vi "LoopselFF.VI"() -> ()   [LabVIEW 2015]
panel:
  in  "alloc mem":bool
  out "FREE \nRAM MB":u64=14006
  out "BUILT-IN\nRAM MB":u64=16662
  out "SEC":dbl=0.06
  out "MB RAM":u64=6
  in  "pos slope":u8=1
  in  "both slopes":u8
  in  "DAT in 10ns":u32
  out "FIFO overflow":bool
  in  "extTrig 0/1":u8
  in  "stop all":bool
  in  "start new block":bool
  in  "Slide":u32(slide)=27666 scale=1.0..3000.0
  in  "frequency[Hz]":u32
  in  "no.of samples (nos)":u32=3000
  in  "exposuretime[ms]":dbl=0.02 format="%.3f"
  out "Signalverlaufgraph":u16[](graph)
  # "Start with run"
  # "Abort with ESC"
  # "1x"
  # "repeat"
  # "exit here"
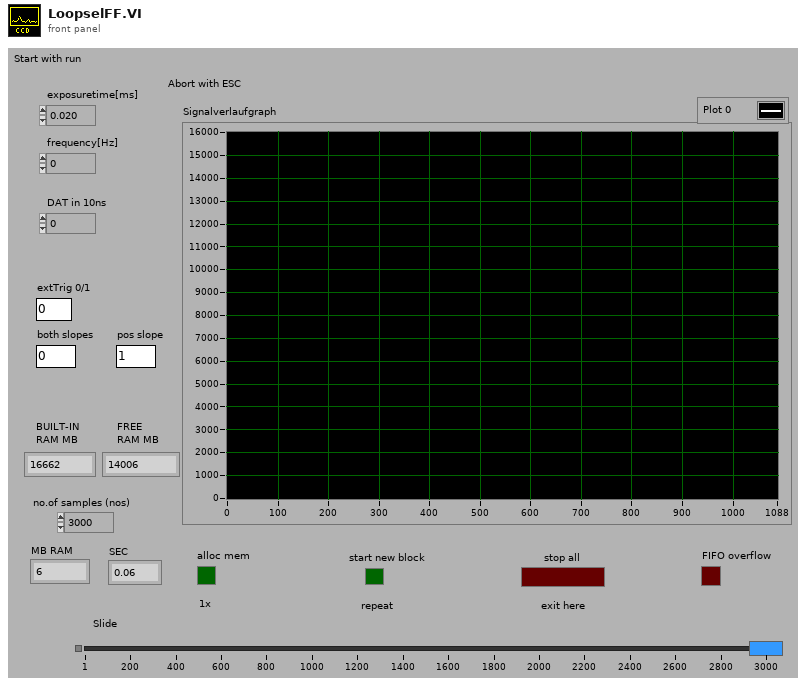
[diagram p1: front panel]
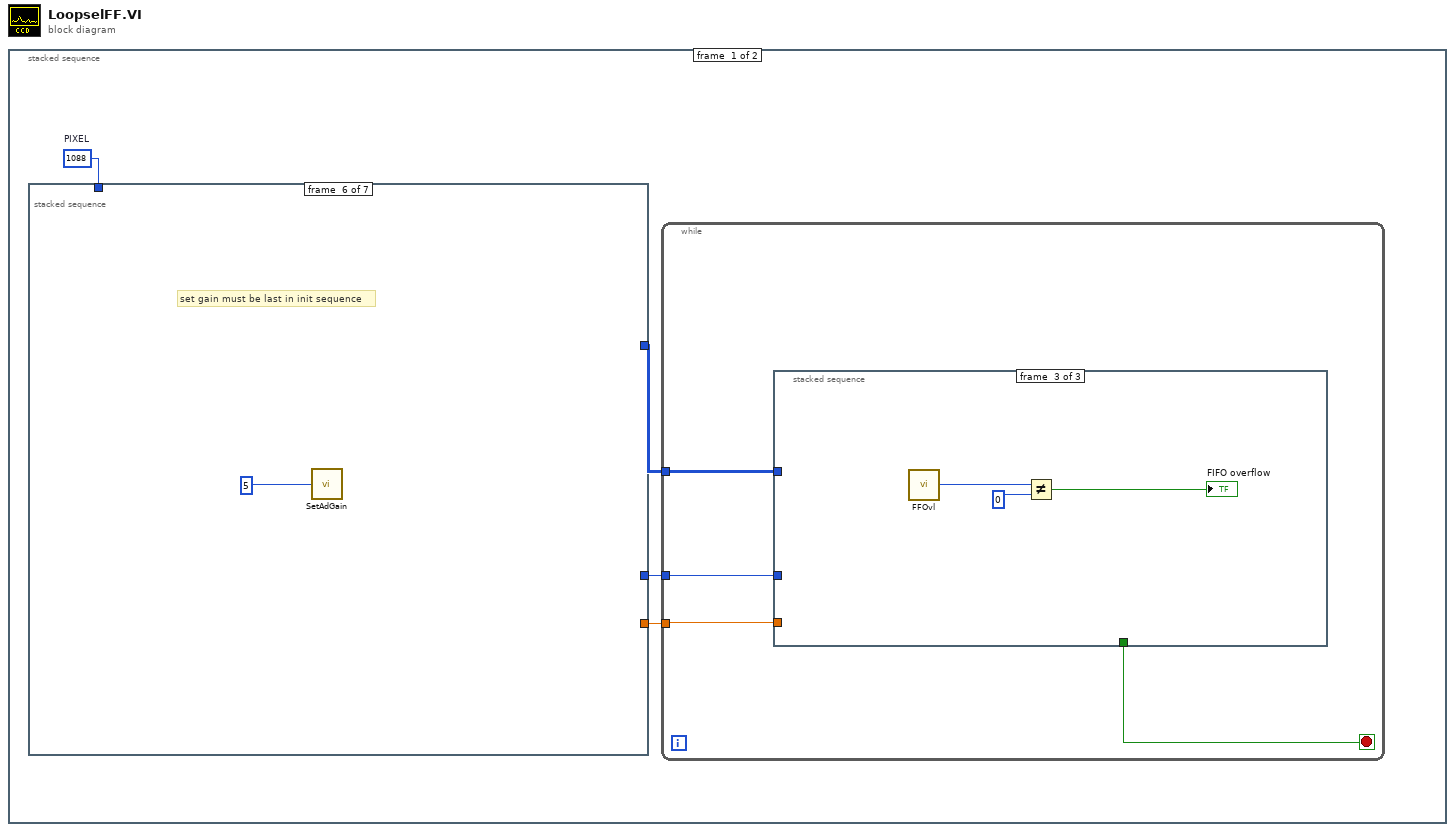
[diagram p0: block diagram]
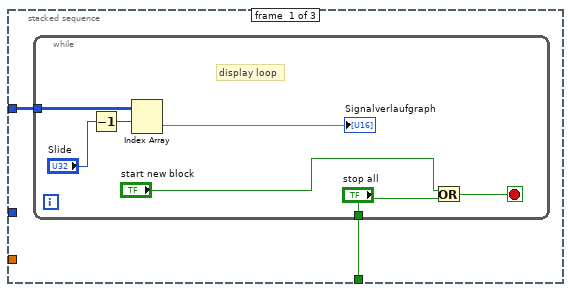
[diagram p2: hidden frame]
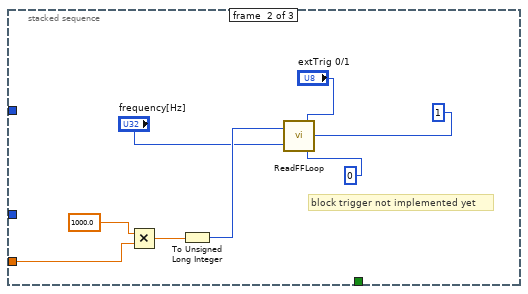
[diagram p3: hidden frame]
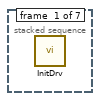
[diagram p4: hidden frame]
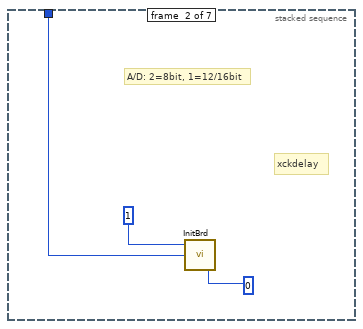
[diagram p5: hidden frame]
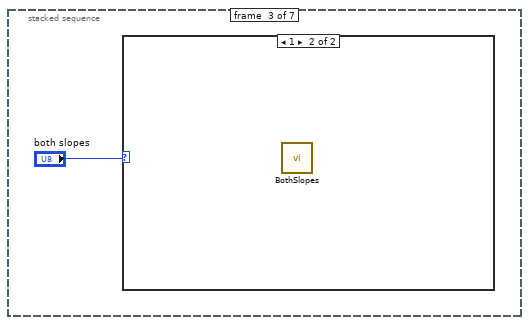
[diagram p6: hidden frame]
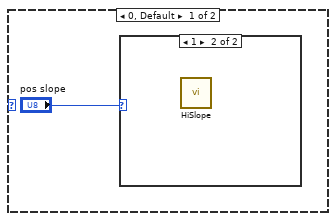
[diagram p7: hidden frame]
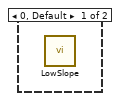
[diagram p8: hidden frame]
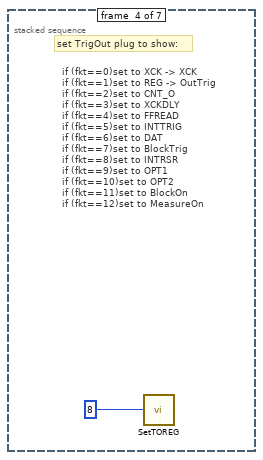
[diagram p9: hidden frame]
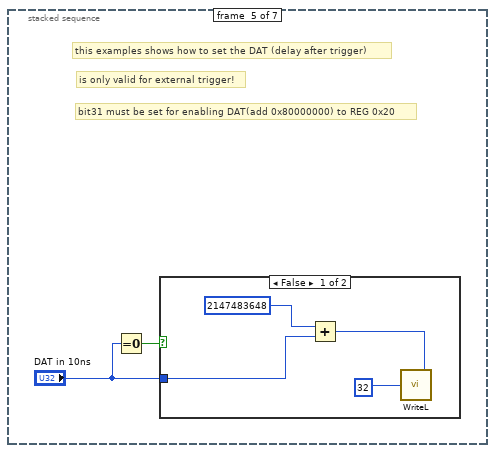
[diagram p10: hidden frame]
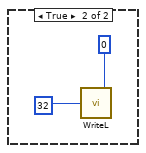
[diagram p11: hidden frame]
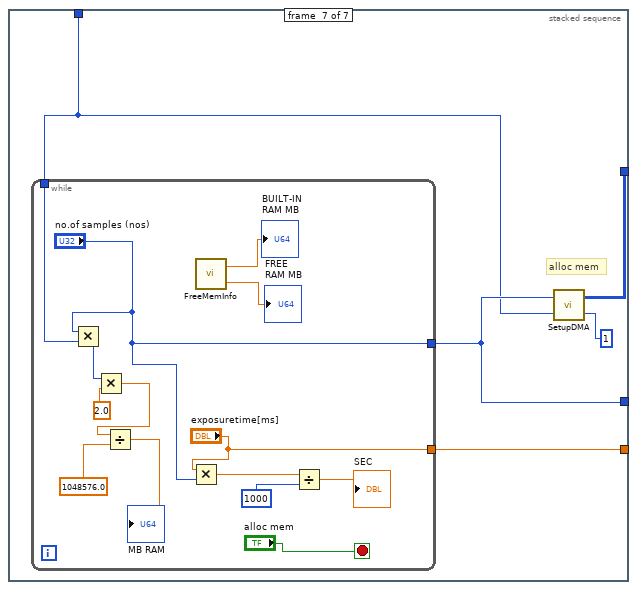
[diagram p12: hidden frame]
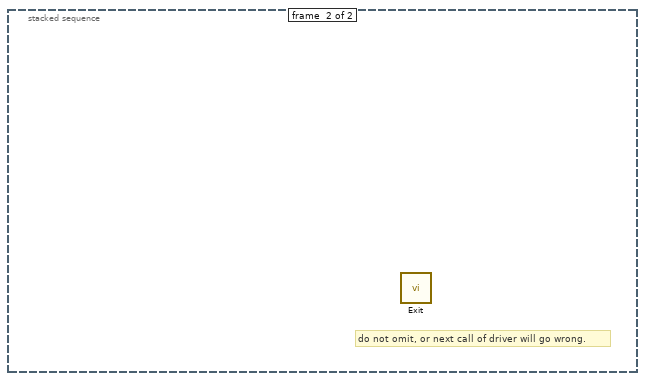
[diagram p13: hidden frame]
diagram:
  n1 = stacked-sequence {
    frame #0 {
      w1 = u32 1088  # PIXEL
      n2 = stacked-sequence {
        tunnel: [_ _ _ _ _ _ w48] -> w4
        tunnel: [_ _ _ _ _ _ w45] -> w3
        tunnel: [_ _ _ _ _ _ w46] -> w2
        tunnel: w1 -> [_ w29 _ _ _ _ w44]
        frame #0 {
          n3 = call "InitDrv.vi"() -> ()  [unwired: 1 in]
        }
        frame #1 {
          # "xckdelay"
          # "A/D: 2=8bit, 1=12/16bit"
          n4 = call "InitBrd.vi"("xckdly"=u32 0, "pixel"=w29, "flag816"=u32 1) -> ()  [unwired: 3 in]
        }
        frame #2 {
          n5 = case shown="1" "both slopes" {
            frame 0, Default {
              n6 = case shown="1" "pos slope" {
                frame 0, Default {
                  n7 = call "LowSlope.vi"() -> ()  [unwired: 1 in]
                }
                frame 1 {
                  n8 = call "HiSlope.vi"() -> ()  [unwired: 1 in]
                }
              }
            }
            frame 1 {
              n9 = call "BothSlopes.vi"() -> ()  [unwired: 1 in]
            }
          }
        }
        frame #3 {
          # "set TrigOut plug to show:"
          # "if (fkt==0)set to XCK -> XCK\nif (fkt==1)set to REG -> OutTrig\nif (fkt==2)set to CNT_O\nif (fkt==3)set to XCKDLY\nif (fkt==4)set to FFREAD\nif (fkt==5)set to INTTRIG\nif (fkt==6)set to DAT\nif (fkt==7)set to BlockTrig\nif (fkt==8)set to INTRSR\nif (fkt==9)set to OPT1\nif (fkt==10)set to OPT2\nif (fkt==11)set to BlockOn\nif (fkt==12)set to MeasureOn"
          n10 = call "SetTOREG.vi"("fkt"=u8 8) -> ()
        }
        frame #4 {
          # "bit31 must be set for enabling DAT(add 0x80000000) to REG 0x20"
          # "is only valid for external trigger!"
          # "this examples shows how to set the DAT (delay after trigger)"
          n11 = Equal To 0?(x="DAT in 10ns") -> (x = 0?=w36:bool)
          n12 = case shown="False" w36 {
            tunnel: "DAT in 10ns" -> [w37 _]
            frame False {
              n13 = Add(x=u32 2147483648, y=w37) -> (x+y=w40:u32)
              n14 = call "WriteL.vi"("val"=w40, "offset"=u32 32) -> ()
            }
            frame True {
              n15 = call "WriteL.vi"("val"=0, "offset"=u32 32) -> ()
            }
          }
        }
        frame #5 {
          # "set gain must be last in init sequence"
          n16 = call "SetAdGain.vi"("gain"=u8 5) -> ()  [unwired: 1 in]
        }
        frame #6 {
          # "alloc mem"
          n17 = while {
            tunnel: w44 -> [w58]
            tunnel: ["exposuretime[ms]"] -> w46
            tunnel: ["no.of samples (nos)"] -> w45
            stop <- "alloc mem" stop-if-true
            n18 = Multiply(x="no.of samples (nos)", y=w58) -> (x*y=w59:u32)
            n19 = Multiply(x=w59, y=2.0) -> (x*y=w60:dbl)
            n20 = Divide(x=w60, y=1048576.0) -> (x/y=→"MB RAM":dbl)
            n21 = Multiply(x="exposuretime[ms]", y="no.of samples (nos)") -> (x*y=w55:dbl)
            n22 = call "FreeMemInfo.vi"() -> ("PhysicalSpace"=→"BUILT-IN\nRAM MB":dbl, "PhysicalFreeSpace"=→"FREE \nRAM MB":dbl)  [unwired: 1 in]
            n23 = Divide(x=w55, y=1000) -> (x/y=→"SEC":dbl)
          }
          n24 = call "SetupDMA.vi"("blocks"=1, "pixel"=w44, "nos"=w45) -> ("Data Values"=w48:u16[][])
        }
      }
      n25 = while {
        tunnel: w4 -> [w8]
        tunnel: w3 -> [w7]
        tunnel: w2 -> [w6]
        stop <- w5 stop-if-true
        n26 = stacked-sequence {
          tunnel: w8 -> [w10 _ _]
          tunnel: w7 -> [_ _ _]
          tunnel: w6 -> [_ w19 _]
          tunnel: [w9 _ _] -> w5
          frame #0 {
            n27 = while {
              tunnel: w10 -> [w15]
              tunnel: ["stop all"] -> w9
              stop <- w13 stop-if-true
              # "display loop"
              n28 = Decrement(x="Slide") -> (x-1=w17:u32)
              n29 = Index Array(array=w15, index (row)=w17) -> (element=→"Signalverlaufgraph":u16[])  [unwired: 1 in]
              n30 = Or(x="start new block", y="stop all") -> (x .or. y?=w13:bool)
            }
          }
          frame #1 {
            # "block trigger not implemented yet"
            n31 = Multiply(x=1000.0, y=w19) -> (x*y=w20:dbl)
            n32 = To Unsigned Long Integer(number=w20) -> (unsigned 32bit integer=w25:u32)
            n33 = call "ReadFFLoop.vi"("exptus"=w25, "freq"="frequency[Hz]", "ExtTrig"="extTrig 0/1", "btrig_ch"=u8 1, "blocktrigger"=u8 0) -> ()
          }
          frame #2 {
            n34 = call "FFOvl.vi"() -> ("FFOvl"=w27:u8)  [unwired: 1 in]
            n35 = Not Equal?(x=w27, y=0) -> (x != y?=→"FIFO overflow":bool)
          }
        }
      }
    }
    frame #1 {
      # "do not omit, or next call of driver will go wrong."
      n36 = call "Exit.vi"() -> ()  [unwired: 1 in]
    }
  }
